vi "Video Stuff v02.vi"() -> ()   [LabVIEW 2009]
doc: "This example illustrates the use of a calibration grid to calibrate and correct an image for nonlinear distortion and accurate shape measurements.\n\nThis example loads the image of a calibration grid used to calibrate the system, learns the grid, then loads an image of parts acquired using the same setup. The example then corrects the image in two ways. The first method corrects the entire image and then measures the area of the coins. The second method corrects only the area of the coins and displays the difference in processing time."
uses:
  <vilib>/userDefined/High Color/IMAQdx.ctl
  <vilib>/vision/NI_Vision_Development_Module.lvlib
  <vilib>/vision/driver/NI_Vision_Acquisition_Software.lvlib
panel:
  out "Transform":T1(plugin-control)
  in  "Camera Name":T2="cam0"
  in  "Video Modes":i32(listbox)
  in  "stop":bool
  out "Live Video":T1(plugin-control)
  out "Buffer Number":u32
  out "Frame Rate":dbl(knob) scale=0.0..100.0 scale format="%.1f"
  in  "Red Range":cluster{"Lower value":i32, "Upper value":i32}={"Lower value"=240, "Upper value"=255}
  in  "Green Range":cluster{"Lower value":i32, "Upper value":i32}={"Lower value"=250, "Upper value"=255}
  in  "Blue Range":cluster{"Lower value":i32, "Upper value":i32}={"Lower value"=250, "Upper value"=255}
  in  "Color Mode":u16(ring) items=["RGB", "HSL", "HSV", "HSI"]
  out "Super Filter":T1(plugin-control)
  in  "Calibration File Path":path=path "C:/Documents and Settings/ekolker/My Documents/OGRE/to be synched/calibrationGrid.PNG"
  out "Top Image":T1(plugin-control) caption="Calibration Template"
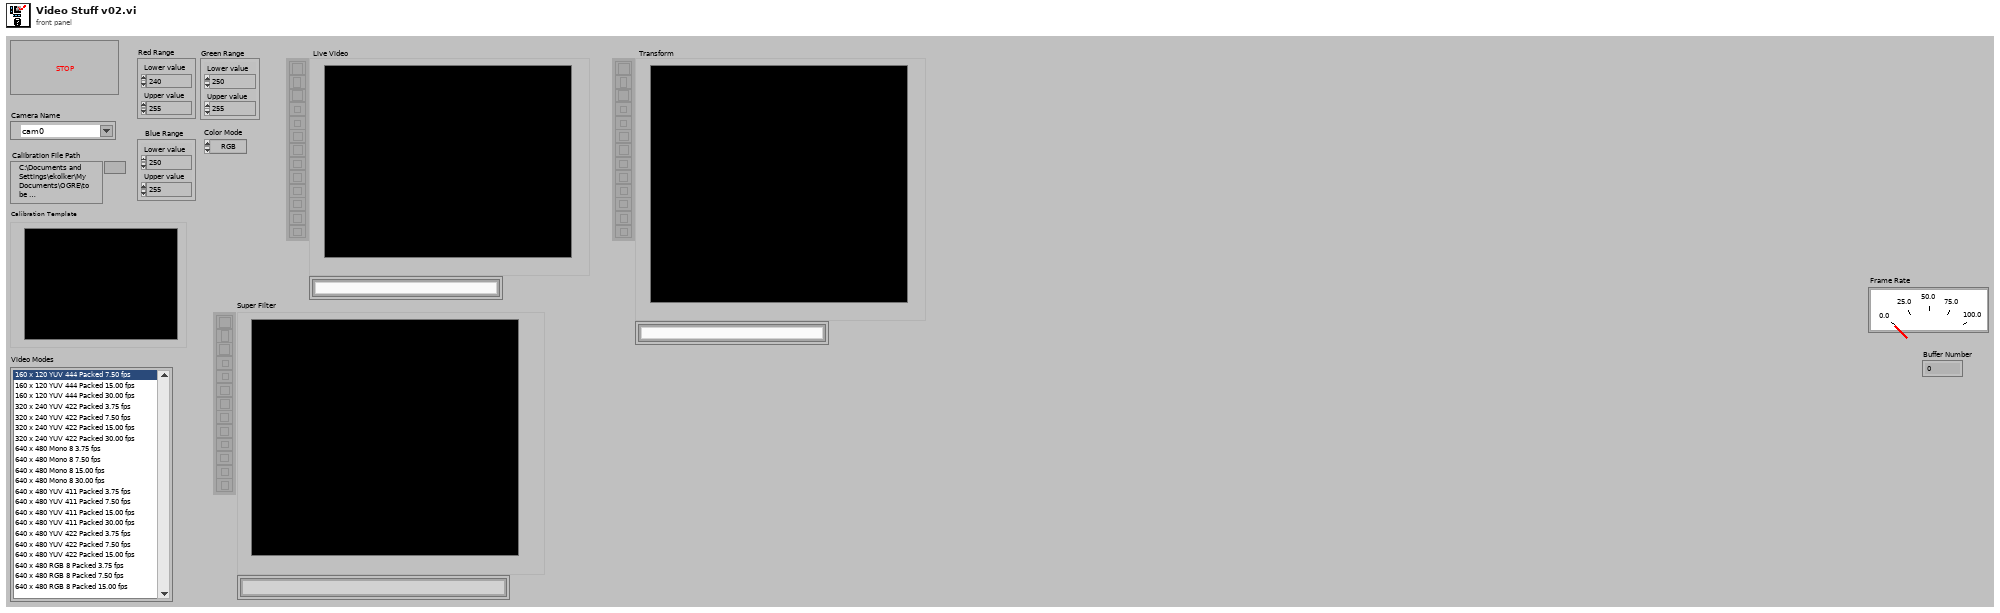
[diagram p1: front panel]
types:
  T1 = typedef "IMAQ Image.ctl" = refnum<image>
  T2 = typedef "IMAQdx.ctl" = refnum<k21>
  T3 = typedef "Image Type" = u32
  T4 = cluster{"X Step":sgl, "Y Step":sgl, "Unit":u32, "Threshold Range":cluster{"Lower value":sgl, "Upper value":sgl}}
  T5 = cluster{"Distortion":u32, "Corrected Image Scaling":u32, "Corrected Image Learn ROI":u32, "Learn Error Map?":bool, "Learn Correction Table?":bool}
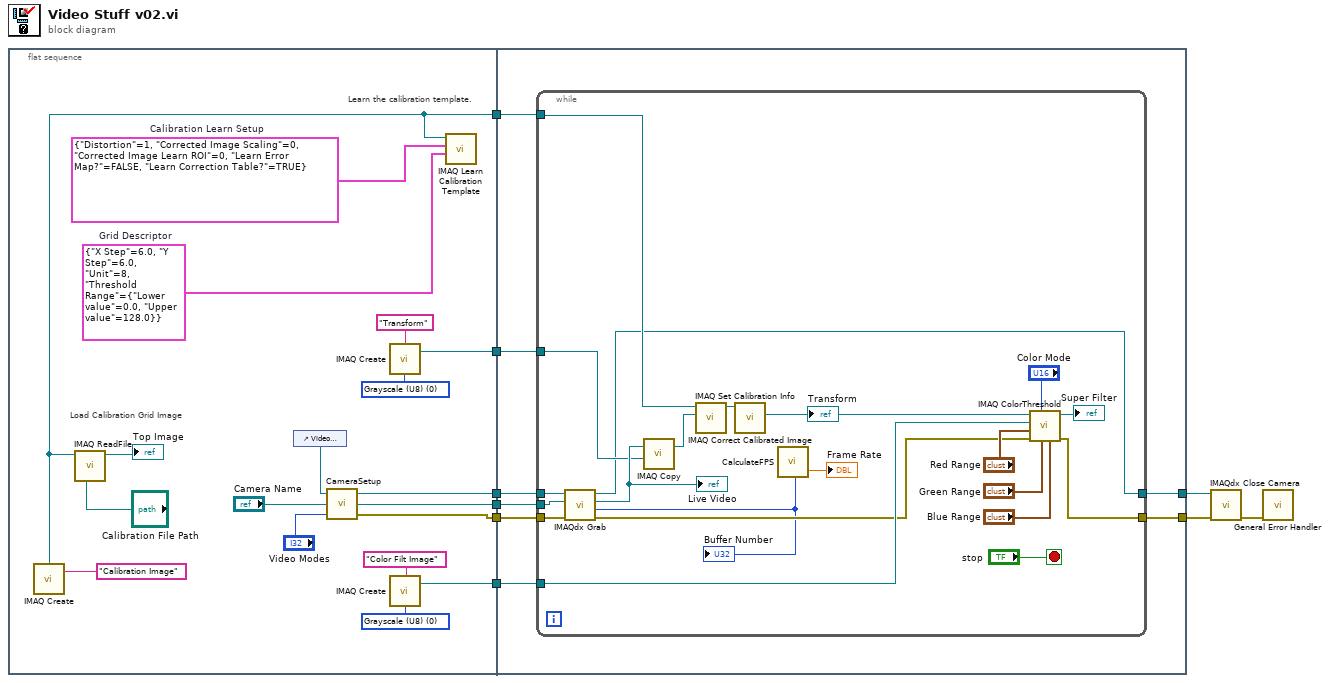
[diagram p0: block diagram]
diagram:
  n1 = flat-sequence {
    tunnel: [w18] -> w9
    tunnel: [w19] -> w5
    tunnel: [w16] -> w4
    tunnel: [w15] -> w3
    tunnel: [w14] -> w2
    tunnel: [w10] -> w1
    tunnel: w9 -> [w35]
    tunnel: [w34] -> w7
    tunnel: [w33] -> w6
    tunnel: w5 -> [w32]
    tunnel: w4 -> [w31]
    tunnel: w3 -> [w30]
    tunnel: w2 -> [w29]
    tunnel: w1 -> [w28]
    frame #0 {
      w12 = T3 0 items=["Grayscale (U8)", "Grayscale (I16)", "Grayscale (SGL)", "Complex (CSG)", "RGB (U32)", "HSL (U32)", "RGB (U64)", "Grayscale (U16)"] ("Image Type")
      w22 = T3 0 items=["Grayscale (U8)", "Grayscale (I16)", "Grayscale (SGL)", "Complex (CSG)", "RGB (U32)", "HSL (U32)", "RGB (U64)", "Grayscale (U16)"] ("Image Type")
      w26 = T4 {"X Step"=6.0, "Y Step"=6.0, "Unit"=8, "Threshold Range"={"Lower value"=0.0, "Upper value"=128.0}}  # Grid Descriptor
      w27 = T5 {"Distortion"=1, "Corrected Image Scaling"=0, "Corrected Image Learn ROI"=0, "Learn Error Map?"=FALSE, "Learn Correction Table?"=TRUE}  # Calibration Learn Setup
      # "Load Calibration Grid Image"
      # "Learn the calibration template."
      n2 = call "IMAQ Create"("Image Name"="Calibration Image") -> ("New Image"=w18:T1)  [unwired: 3 in, 2 out]
      n3 = call "IMAQ ReadFile"("File Path"="Calibration File Path", "Image"=w18) -> ("Image Out"=→"Top Image":T1)  [unwired: 3 in, 6 out]
      n4 = control-ref of="Video Modes"() -> (w13:refnum<vi>)
      n5 = call "CameraSetup.vi"("Video Modes"="Video Modes", "Camera Name"="Camera Name", "reference"=w13) -> ("error out"=w14:errorcluster, "New Image"=w15:T1, "Session Out"=w16:T2)
      n6 = call "IMAQ Create"("Image Name"="Transform", "Image Type"=w12) -> ("New Image"=w10:T1)  [unwired: 2 in, 2 out]
      n7 = call "IMAQ Create"("Image Name"="Color Filt Image", "Image Type"=w22) -> ("New Image"=w19:T1)  [unwired: 2 in, 2 out]
      n8 = call "IMAQ Learn Calibration Template"("Grid Descriptor"=w26, "Calibration Learn Setup"=w27, "Image"=w18) -> ()  [unwired: 4 in, 5 out]
    }
    frame #1 {
      n9 = while {
        tunnel: w35 -> [w41]
        tunnel: w32 -> [w56]
        tunnel: [w37] -> w34
        tunnel: [w36] -> w33
        tunnel: w31 -> [w46]
        tunnel: w30 -> [w45]
        tunnel: w29 -> [w44]
        tunnel: w28 -> [w39]
        stop <- "stop" stop-if-true
        n10 = call <vilib>:"IMAQdx Grab.vi"("error in"=w44, "Image In"=w45, "Session In"=w46) -> ("error out"=w48:errorcluster, "Buffer Number Out"=w47:u32, "Image Out"=w43:T1, "Session Out"=w37:T2)  [unwired: 1 in, 4 out]
        "Live Video" <- w43
        "Buffer Number" <- w47
        n11 = call "IMAQ Copy"("Image Dst"=w39, "Image Src"=w43) -> ("Image Dst Out"=w42:T1)  [unwired: 4 in, 1 out]
        n12 = call "IMAQ Set Calibration Info"("Image Dst"=w42, "Image Src"=w41) -> ("Calibrated Image"=w40:T1)  [unwired: 2 in, 7 out]
        n13 = call "IMAQ Correct Calibrated Image"("Image Src"=w40) -> ("Corrected Image"=w38:T1)  [unwired: 6 in, 4 out]
        "Transform" <- w38
        n14 = call "CalculateFPS.vi"("buffer number"=w47) -> ("processed FPS"=→"Frame Rate":dbl)  [unwired: 2 out]
        n15 = call "IMAQ ColorThreshold"("Blue or Luma or Val or Inten Range"="Blue Range", "Green or Sat Range"="Green Range", "Color Mode"="Color Mode", "error in (no error)"=w48, "Red or Hue Range"="Red Range", "Image Dst"=w56, "Image Src"=w38) -> ("error out"=w36:errorcluster, "Image Dst Out"=→"Super Filter":T1)  [unwired: 3 in]
      }
    }
  }
  n16 = call <vilib>:"IMAQdx Close Camera.vi"("error in"=w6, "Session In"=w7) -> ("error out"=w8:errorcluster)  [unwired: 9 out]
  n17 = call <vilib>:"General Error Handler.vi"("error in (no error)"=w8) -> ()  [unwired: 1 in, 14 out]
